vi "ep_Read Wiring.vi"(8 "error in (no error)":errorcluster, 11 "system info in":refnum<class "EP System Info.lvclass">) -> (0 "error out":errorcluster, 1 "line voltage?":bool, 2 "wiring":T1=enum."3xUph + 4xI", 3 "system info out":refnum<class "EP System Info.lvclass">)   [LabVIEW 2011, in "NI_EP_Power Quality.lvlib" / "EP System Info.lvclass"]
uses:
  <vilib>/addons/Electrical Power/PQ/Common/Classes/System Info/EP System Info.lvclass
  <vilib>/addons/Electrical Power/PQ/Common/Controls/ep_Wiring.ctl
  <vilib>/addons/Electrical Power/PQ/Common/Classes/System Info/EP System Info.lvclass/EP System Info.ctl
  <vilib>/addons/Electrical Power/PQ/NI_EP_Power Quality.lvlib
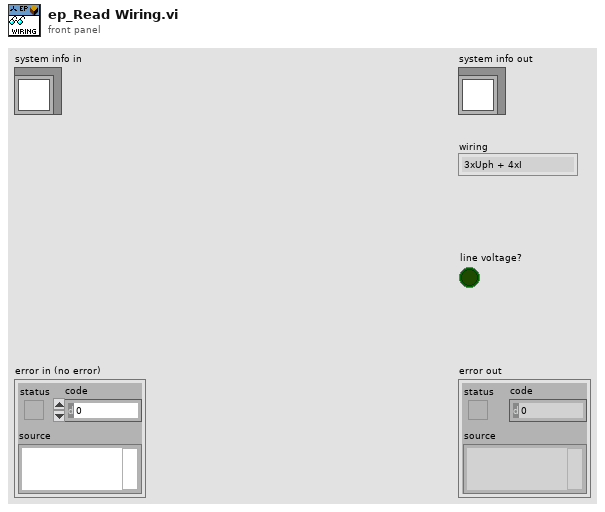
[diagram p1: front panel]
types:
  T1 = typedef "NI_EP_Power Quality.lvlib/ep_Wiring.ctl" = enum16{"4xUph + 4xI", "3xUph + 4xI", "3xUline + 4xI", "3xUph + 3xI", "3xUline + 3xI", "3xUph + 2xI", "3xUline + 2xI", "1xUph + 1xI"}
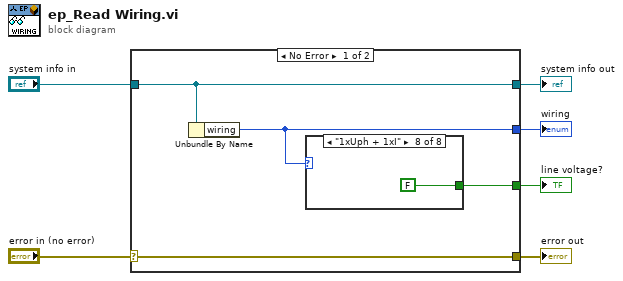
[diagram p0: block diagram]
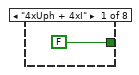
[diagram p2: hidden frame]
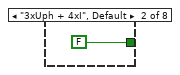
[diagram p3: hidden frame]
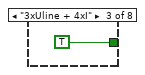
[diagram p4: hidden frame]
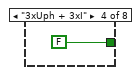
[diagram p5: hidden frame]
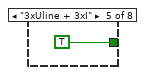
[diagram p6: hidden frame]
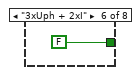
[diagram p7: hidden frame]
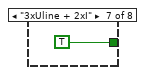
[diagram p8: hidden frame]
diagram:
  n1 = case shown="No Error" "error in (no error)" {
    selector: "error in (no error)" -> [w10 w19]
    tunnel: [w10 w19] -> w5
    tunnel: [w9 w20] -> w3
    tunnel: "system info in" -> [w9 w20]
    tunnel: [w8 _] -> w2
    tunnel: [w7 _] -> w1
    frame No Error {
      n2 = Unbundle By Name(w9) -> ("wiring"=w8:T1)
      n3 = case shown="\"1xUph + 1xI\"" w8 {
        tunnel: [FALSE FALSE TRUE FALSE TRUE FALSE TRUE FALSE] -> w7
        frame "4xUph + 4xI" {
        }
        frame "3xUph + 4xI", Default {
        }
        frame "3xUline + 4xI" {
        }
        frame "3xUph + 3xI" {
        }
        frame "3xUline + 3xI" {
        }
        frame "3xUph + 2xI" {
        }
        frame "3xUline + 2xI" {
        }
        frame "1xUph + 1xI" {
        }
      }
    }
    frame Error {
    }
  }
  "error out" <- w5
  "system info out" <- w3
  "wiring" <- w2
  "line voltage?" <- w1
